vi "Letter Statistics Any Sort.vi"(11 "Statistic in":T1[](array[typedef])) -> (3 "Statistic out":T1[](array[typedef]))   [LabVIEW 2015]
uses:
  TypeDef/Letter Statistic.ctl
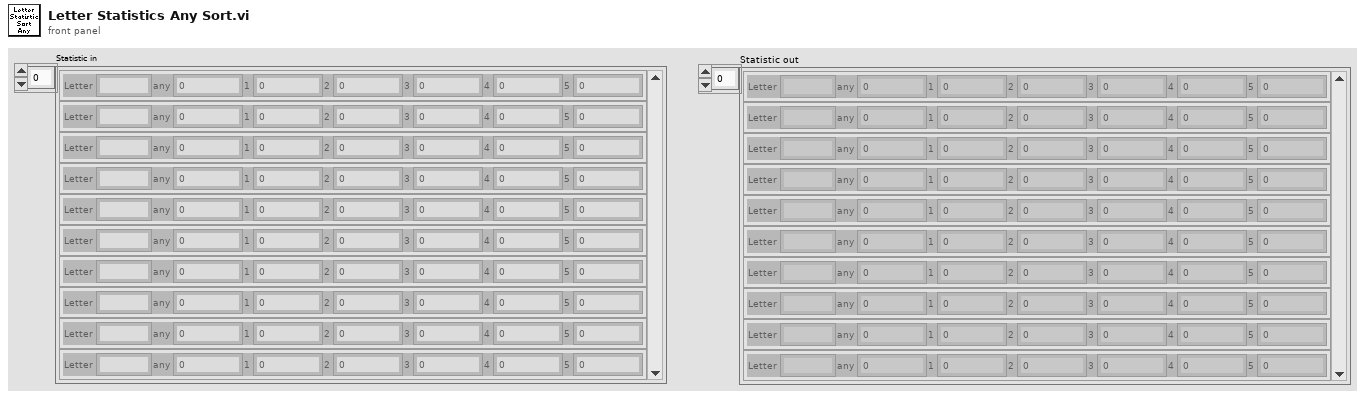
[diagram p1: front panel]
types:
  T1 = typedef "Letter Statistic.ctl" = cluster{"Letter":string, "any":dbl, "1":dbl, "2":dbl, "3":dbl, "4":dbl, "5":dbl}
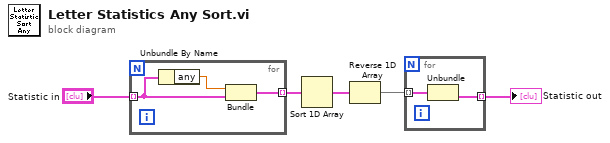
[diagram p0: block diagram]
diagram:
  n1 = for {
    tunnel: "Statistic in" -> [w8] mode=indexing
    tunnel: [w6] -> w4 mode=indexing
    n2 = Unbundle By Name(w8) -> ("any"=w7:dbl)
    n3 = Bundle("any"=w7, "Letter Statistic"=w8) -> (w6:cluster{"any":dbl, "Letter Statistic":T1})  [unwired: 1 in]
  }
  n4 = Sort 1D Array(array=w4) -> (sorted array=w3:cluster{"any":dbl, "Letter Statistic":T1}[])
  n5 = Reverse 1D Array(array=w3) -> (reversed array=w2:cluster{"any":dbl, "Letter Statistic":T1}[])
  n6 = for {
    tunnel: w2 -> [w10] mode=indexing
    tunnel: [w9] -> w1 mode=indexing
    n7 = Unbundle(w10) -> ("Letter Statistic"=w9:T1)  [unwired: 1 out]
  }
  "Statistic out" <- w1
